vi "updateSettings.vi"(8 "error in (no error)":errorcluster, 9 "ID":u32, 10 "Serial Number":string, 11 "Calibrador in":refnum<class "Calibrador.lvclass">) -> (0 "error out":errorcluster, 3 "Calibrador out":refnum<class "Calibrador.lvclass">)   [LabVIEW 2019, in "Calibrador.lvclass"]
uses:
  Calibrador.lvclass
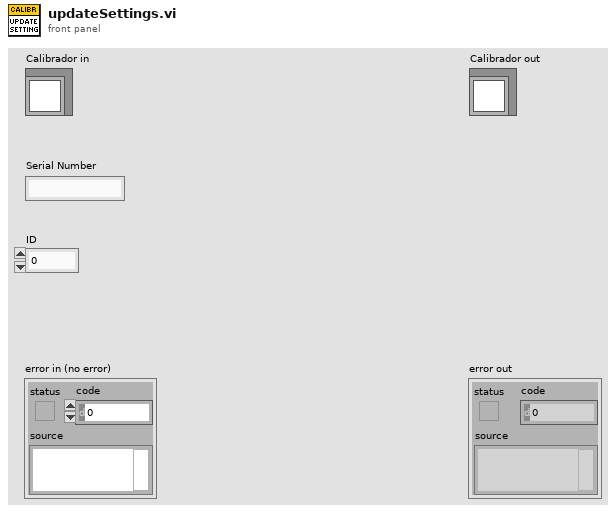
[diagram p1: front panel]
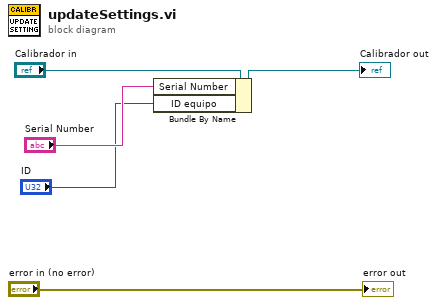
[diagram p0: block diagram]
diagram:
  n1 = Bundle By Name(cluster="Calibrador in", "Serial Number"="Serial Number", "ID equipo"="ID") -> (→"Calibrador out":refnum<class "Calibrador.lvclass">)
  "error out" <- "error in (no error)"
